vi "Initialize Hamburger.vi"(8 "error in (no error)":errorcluster, 10 "MenuVI Path":path) -> (0 "error out":errorcluster, 2 "HamburgerItemClicked Event":refnum<user-event>, 3 "HamburgerMenu Obj":refnum<class "HamburgerMenu.lvclass">)   [LabVIEW 2017, in "Hamburger Menu Library.lvlib" / "HamburgerMenu.lvclass"]
uses:
  HamburgerMenu.lvclass
  HamburgerMenu.lvclass/HamburgerMenu.ctl
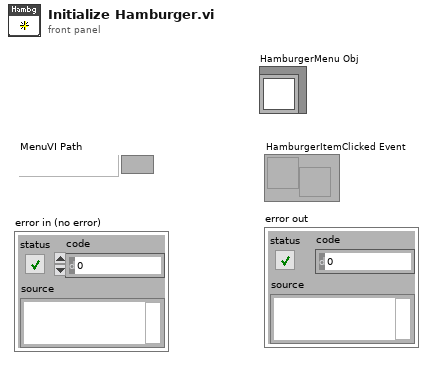
[diagram p1: front panel]
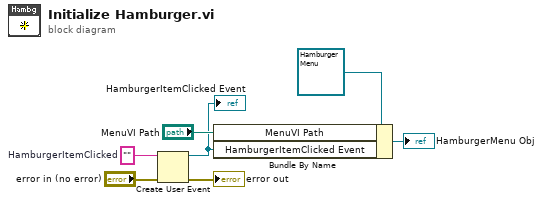
[diagram p0: block diagram]
diagram:
  w7 = ""  # HamburgerItemClicked
  n1 = Create User Event(user event datatype=w7, error in="error in (no error)") -> (user event=w1:refnum<user-event>, error out=→"error out":errorcluster)
  "HamburgerItemClicked Event" <- w1
  n2 = Bundle By Name(cluster=refnum<class "HamburgerMenu.lvclass"> refnum ("HamburgerMenu Obj"), "MenuVI Path"="MenuVI Path", "HamburgerItemClicked Event"=w1) -> (→"HamburgerMenu Obj":refnum<class "HamburgerMenu.lvclass">)
